vi "Get Homed Status.vi"(8 "error in (no error)":errorcluster, 11 "Axis in":refnum<class "Axis.lvclass">) -> (0 "error out":errorcluster, 2 "Homed?":bool, 3 "Axis out":refnum<class "Axis.lvclass">)   [LabVIEW 2018, in "Axis.lvlib" / "Axis.lvclass"]
uses:
  Axis.lvclass
  Custom Controls/Command.ctl
  Axis.lvclass/Axis.ctl
  Axis.lvlib
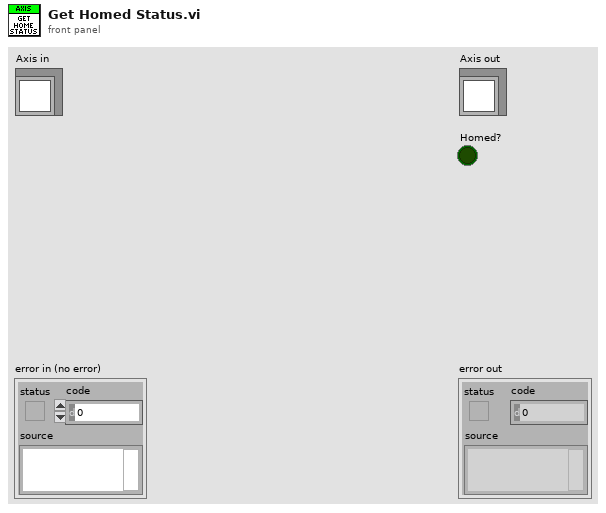
[diagram p1: front panel]
types:
  T1 = typedef "Axis.lvlib/Command.ctl" = enum16{"None", "Home", "Renumber", "Move Absolute", "Move Relative", "Stop", "Set Run Speed", "Set Acceleration", "Set Run Current", "Set Home Offset", "Set Home Speed", "Query Current Position", "Load Defaults", "Query Status", "Lock Controls", "Unlock Controls", "Set Jog Step Size", "Set Jog Acceleration", "Set Jog Speed", "Query Homed Status", "Query Moving Status", "Reset", "Set Max Position", "Set Min Position"}
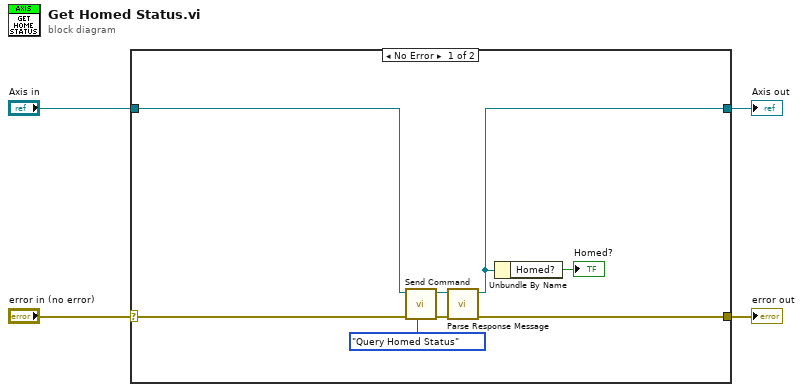
[diagram p0: block diagram]
diagram:
  n1 = case shown="No Error" "error in (no error)" {
    selector: "error in (no error)" -> [w8 w14]
    tunnel: [w7 w14] -> w3
    tunnel: [w5 w13] -> w1
    tunnel: "Axis in" -> [w6 w13]
    frame No Error {
      n2 = call-dynamic "Send Command.vi"("Command"=Command."Query Homed Status", "error in"=w8, "Axis in"=w6) -> ("error out"=w10:errorcluster, "Axis out"=w11:refnum<class "Axis.lvclass">)  [unwired: 7 in]
      n3 = call-dynamic "Parse Response Message.vi"("error in"=w10, "Axis in"=w11) -> ("error out"=w7:errorcluster, "Axis out"=w5:refnum<class "Axis.lvclass">)  [unwired: 8 in]
      n4 = Unbundle By Name(w5) -> ("Homed?"=→"Homed?":bool)
    }
    frame Error {
    }
  }
  "error out" <- w3
  "Axis out" <- w1
